vi "Set Attribute Tree Data.vi"(7 "Tree ID":string, 8 "Error In":errorcluster, 9 "Attribute Value":refnum<class "Tree Data.lvclass">, 10 "Attribute Name":string, 11 "Tree Manager":T1) -> (0 "Error Out":errorcluster, 1 "Replaced?":bool, 3 "Tree Manager":T1)   [LabVIEW 2016, in "Tree Manager.lvclass"]
doc: "Set a Tree Data object as an attribute of the Tree."
uses:
  Tree Manager.lvclass
  Typedefs/Session Handle.ctl
  Tree Data/Tree Data.lvclass
  Tree Manager.lvclass/Tree Manager.ctl
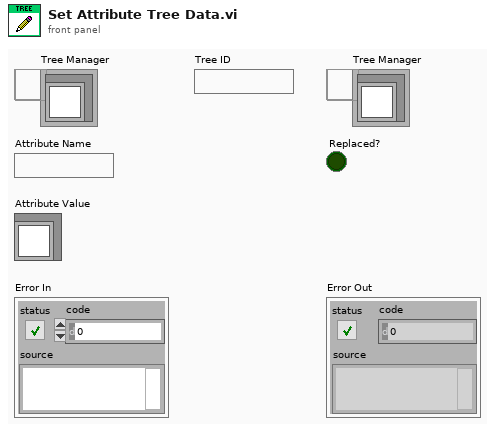
[diagram p1: front panel]
types:
  T1 = typedef "Tree Manager.lvclass/Session Handle.ctl" = refnum<data-value>
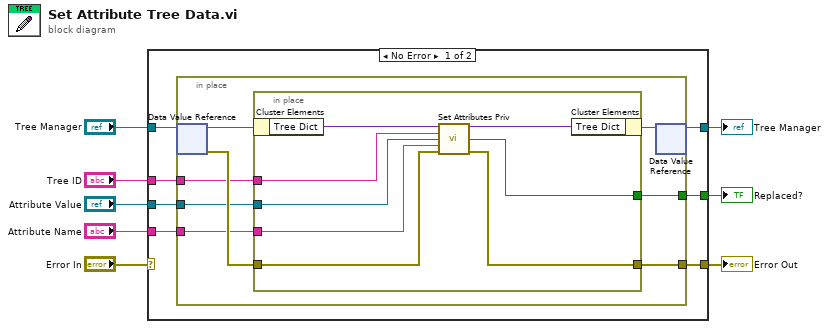
[diagram p0: block diagram]
diagram:
  n1 = case shown="No Error" "Error In" {
    selector: "Error In" -> [_ w32]
    tunnel: "Tree Manager" -> [w15 w33]
    tunnel: [w14 w33] -> w7
    tunnel: [w13 w32] -> w5
    tunnel: "Tree ID" -> [w12 _]
    tunnel: "Attribute Value" -> [w11 _]
    tunnel: "Attribute Name" -> [w10 _]
    tunnel: [w9 _] -> w2
    frame No Error {
      n2 = in-place {
        in-place-border: [w22] -> w13
        in-place-border: w12 -> [w19]
        in-place-border: w11 -> [w18]
        in-place-border: w10 -> [w17]
        in-place-border: [w16] -> w9
        n3 = in-place-dvr #1(w15) -> (w23:refnum<class "Tree Manager.lvclass">, w20:errorcluster)
        n4 = in-place {
          in-place-border: [w25] -> w22
          in-place-border: w20 -> [w26]
          in-place-border: w19 -> [w29]
          in-place-border: w18 -> [w28]
          in-place-border: w17 -> [w27]
          in-place-border: [w24] -> w16
          n5 = in-place-cluster #2(w23) -> ("Tree Dict"=w31:variant)
          n6 = call "Set Attributes Priv.vi"("Tree Dictionary Out"=w31, "Unique ID"=w29, "Data"=w28, "Name"=w27, "error in"=w26) -> ("Tree Dictionary Out"=w30:variant, "Replaced?"=w24:bool, "error out"=w25:errorcluster)  [unwired: 8 in]
          n7 = in-place-cluster #2("Tree Dict"=w30) -> (w21:refnum<class "Tree Manager.lvclass">)
        }
        n8 = in-place-dvr #1(w21) -> (w14:T1)  [unwired: 1 out]
      }
    }
    frame Error {
    }
  }
  "Tree Manager" <- w7
  "Error Out" <- w5
  "Replaced?" <- w2
